vi "Test A.vi"() -> ()   [LabVIEW 2023, in "LabGRAD.lvlib"]
uses:
  LabGRAD.lvlib
  Value/Value.lvclass
  UiObjects/numeric value control.ctl
  Value/Value.lvclass/Value.ctl
  Value/multiply value.vi
  Value/add float.vi
  Value/power float.vi
  UiObjects/UiObjects.lvclass
  UiObjects/string control.ctl
panel:
  out "grad":T1
  out "Value 2":T1
  in  "LabGRAD.lvlib:Value.lvclass":refnum<class "Value.lvclass">
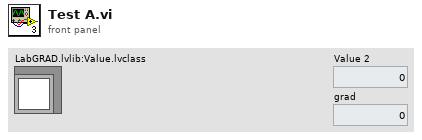
[diagram p1: front panel]
types:
  T1 = typedef "UiObjects.lvlib/UiObjects.lvclass/numeric value control.ctl" = dbl
  T2 = typedef "UiObjects.lvlib/UiObjects.lvclass/string control.ctl" = string
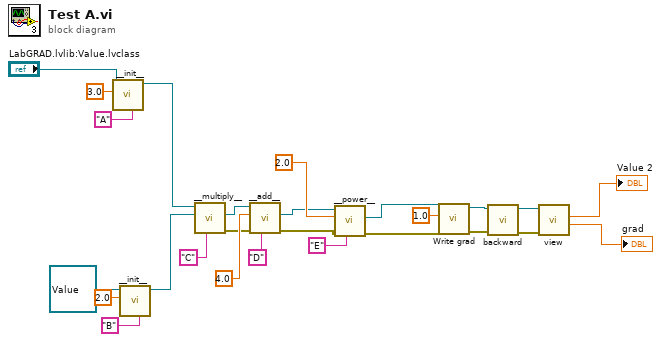
[diagram p0: block diagram]
diagram:
  n1 = call "__init__.vi"("Label"=T2 "A", "data"=T1 3.0, "Value in"="LabGRAD.lvlib:Value.lvclass") -> ("Value out"=w10:refnum<class "Value.lvclass">)  [unwired: 7 in, 1 out]
  n2 = call "__init__.vi"("Label"=T2 "B", "data"=T1 2.0, "Value in"=refnum<class "Value.lvclass"> refnum ("LabGRAD.lvlib:Value.lvclass")) -> ("Value out"=w15:refnum<class "Value.lvclass">)  [unwired: 7 in, 1 out]
  n3 = call-poly "__multiply__.vi"("label"=T2 "C", "B"=w15, "A"=w10) -> ("error out"=w13:errorcluster, "C"=w14:refnum<class "Value.lvclass">)  [unwired: 6 in, 1 out]
  n4 = call-poly "__add__.vi"("label"=T2 "D", "i"=w13, "B"=T1 4.0, "A"=w14) -> ("error out"=w12:errorcluster, "c"=w11:refnum<class "Value.lvclass">)  [unwired: 5 in, 1 out]
  n5 = call-poly "__power__.vi"("label"=T2 "E", "error in (no error)"=w12, "B"=T1 2.0 ("Value"), "A"=w11) -> ("error out"=w17:errorcluster, "C"=w16:refnum<class "Value.lvclass">)  [unwired: 5 in, 1 out]
  n6 = call "Write grad.vi"("error in (no error)"=w17, "Numeric"=T1 1.0, "Value in"=w16) -> ("error out"=w9:errorcluster, "Value out"=w8:refnum<class "Value.lvclass">)  [unwired: 7 in]
  n7 = call "backward.vi"("error in (no error)"=w9, "Value in"=w8) -> ("error out"=w7:errorcluster, "Value out"=w6:refnum<class "Value.lvclass">)  [unwired: 8 in]
  n8 = call "view.vi"("error in (no error)"=w7, "Value in"=w6) -> ("grad"=→"grad":T1, "Value"=→"Value 2":T1)  [unwired: 5 in, 3 out]
